vi "Init Tx - Data.vi"(7 "Data Access in":refnum<class "Data Access Engine.lvclass">, 8 "error in (no error)":errorcluster, 11 "Parameters":variant) -> (0 "error out":errorcluster, 3 "Tx Loop Data":T1, 5 "Data Access out":refnum<class "Data Access Engine.lvclass">)   [LabVIEW 2016, in "UDP-Custom-Device Engine.lvlib"]
uses:
  UDP-Custom-Device Engine.lvlib
  <vilib>/NI/NIVS Inline Async API/_Data Access Engine/Data Access Engine/Data Access Engine.lvclass
  Types/Engine - Tx Loop Data.ctl
  <vilib>/NI Veristand/VeriStand Data/Library/Byte Buffer/Byte Buffer.lvclass
  <vilib>/NI/NIVS Inline Async API/_Data Access Engine/Data Access Engine/Types/Read.DVR.ctl
  <vilib>/NI/NIVS Inline Async API/_Data Access Engine/Access Type Classes/Read/Read.lvclass
  <vilib>/NI Veristand/VeriStand Data/Library/Typedefs/Typedefs.Data Types.ctl
  Types/Engine - Data Conversion Config.ctl
  <vilib>/NI Veristand/VeriStand Data/Library/Byte Buffer/Byte Buffer.Mapping.ctl
  Shared/Types/Shared - Header Details.ctl
  Shared/Types/Shared - Tx.PacketInfo.ctl
  Shared/Types/Shared - Channel Data Type.ctl
  Shared/Types/Shared - Buffered.PacketInfo.ctl
  <vilib>/NI/NIVS Inline Async API/_Data Access Engine/Data Access Engine/Methods/Read.Lookup.vi
  Shared/UDP-Custom-Device Shared.lvlib
  <vilib>/NI Veristand/VeriStand Data/Library/VeriStand Data.lvlib
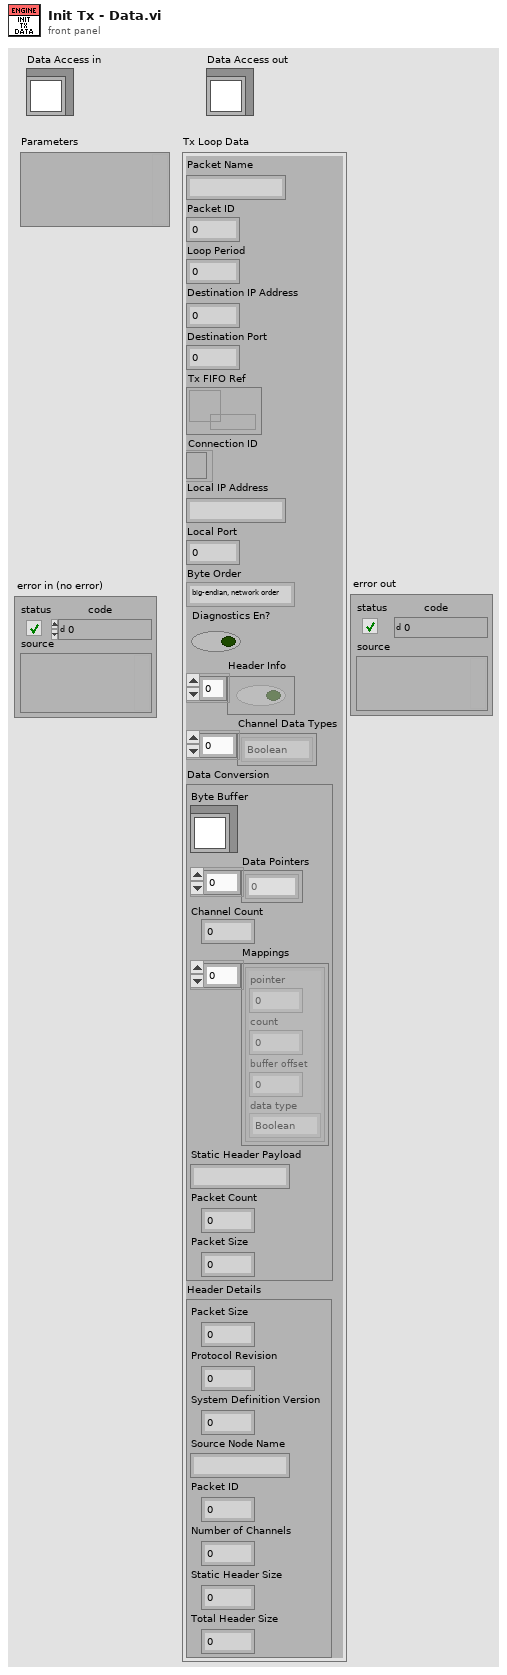
[diagram p1: front panel]
types:
  T1 = typedef "UDP-Custom-Device Engine.lvlib/Engine - Tx Loop Data.ctl" = cluster{"Packet Name":string, "Packet ID":i32, "Loop Period":u32, "Destination IP Address":u32, "Destination Port":u16, "Tx FIFO Ref":T2, "Connection ID":refnum<k16>, "Local IP Address":string, "Local Port":i32, "Byte Order":enum16{"big-endian, network order", "native, host order", "little-endian"}, "Diagnostics En?":bool, "Header Info":bool[], "Channel Data Types":T3[], "Data Conversion":T4, "Header Details":T6}
  T2 = typedef "Data Access Engine.lvlib/Data Access Engine.lvclass/Read.DVR.ctl" = refnum<data-value>
  T3 = typedef "VeriStand Data.lvlib/Typedefs.Data Types.ctl" = enum16{"Boolean", "Single", "Double", "I8", "I16", "I32", "I64", "U8", "U16", "U32", "U64"}
  T4 = typedef "UDP-Custom-Device Engine.lvlib/Engine - Data Conversion Config.ctl" = cluster{"Byte Buffer":refnum<class "Byte Buffer.lvclass">, "Data Pointers":u64[], "Channel Count":i32, "Mappings":T5[], "Static Header Payload":string, "Packet Count":dbl, "Packet Size":i32}
  T5 = typedef "VeriStand Data.lvlib/Byte Buffer.lvclass/Byte Buffer.Mapping.ctl" = cluster{"pointer":u64, "count":i32, "buffer offset":i32, "data type":T3}
  T6 = typedef "UDP-Custom-Device Shared.lvlib/Shared - Header Details.ctl" = cluster{"Packet Size":u16, "Protocol Revision":u8, "System Definition Version":u64, "Source Node Name":string, "Packet ID":u32, "Number of Channels":u32, "Static Header Size":u16, "Total Header Size":u16}
  T7 = typedef "UDP-Custom-Device Shared.lvlib/Shared - Tx.PacketInfo.ctl" = cluster{"Packet Name":string, "Packet ID":i32, "Decimation":u16, "Destination IP Address":string, "Destination Port":u16, "Local IP Address":string, "Local Port":u16, "Endianness":u16, "Diagnostics En?":bool, "Header Info":bool[], "PCL Period":u32, "Channel Data Types":T8[], "Header Details":T6, "Buffered Packet Info":T9}
  T8 = typedef "UDP-Custom-Device Shared.lvlib/Shared - Channel Data Type.ctl" = enum16{"Boolean", "Single", "Double", "I8", "I16", "I32", "I64", "U8", "U16", "U32", "U64"}
  T9 = typedef "UDP-Custom-Device Shared.lvlib/Shared - Buffered.PacketInfo.ctl" = cluster{"Buffer Size":u32, "External Buffer":bool, "Prepend Header":bool, "Is Buffered":bool}
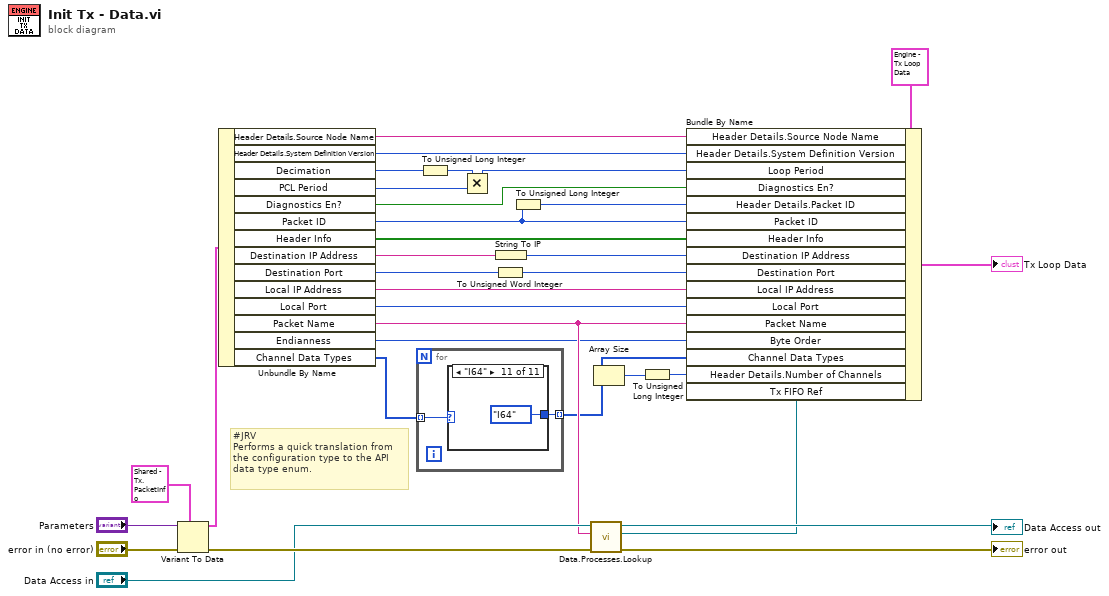
[diagram p0: block diagram]
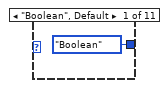
[diagram p2: hidden frame]
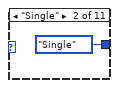
[diagram p3: hidden frame]
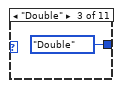
[diagram p4: hidden frame]
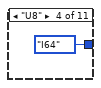
[diagram p5: hidden frame]
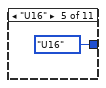
[diagram p6: hidden frame]
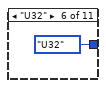
[diagram p7: hidden frame]
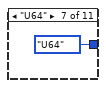
[diagram p8: hidden frame]
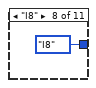
[diagram p9: hidden frame]
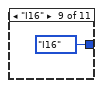
[diagram p10: hidden frame]
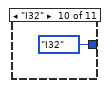
[diagram p11: hidden frame]
diagram:
  # "#JRV\nPerforms a quick translation from\nthe configuration type to the API\ndata type enum."
  n1 = Variant To Data(error in="error in (no error)", type=T7 {"Packet Name"="", "Packet ID"=0, "Decimation"=0, "Destination IP Address"="", "Destination Port"=0, "Local IP Address"="", "Local Port"=0, "Endianness"=0, "Diagnostics En?"=FALSE, "Header Info"=[], "PCL Period"=0, "Channel Data Types"=[], "Header Details"={"Packet Size"=0, "Protocol Revision"=0, "System Definition Version"=0, "Source Node Name"="", "Packet ID"=0, "Number of Channels"=0, "Static Header Size"=0, "Total Header Size"=0}, "Buffered Packet Info"={"Buffer Size"=0, "External Buffer"=FALSE, "Prepend Header"=FALSE, "Is Buffered"=FALSE}} ("Packet Info"), Variant="Parameters") -> (data=w31:T7, error out=w30:errorcluster)
  n2 = Unbundle By Name(w31) -> ("Header Details.Source Node Name"=w2:string, "Header Details.System Definition Version"=w1:u64, "Decimation"=w15:u16, "PCL Period"=w16:u32, "Diagnostics En?"=w18:bool, "Packet ID"=w8:i32, "Header Info"=w17:bool[], "Destination IP Address"=w10:string, "Destination Port"=w12:u16, "Local IP Address"=w22:string, "Local Port"=w21:u16, "Packet Name"=w23:string, "Endianness"=w19:u16, "Channel Data Types"=w13:T8[])
  n3 = for {
    tunnel: w13 -> [w35] mode=indexing
    tunnel: [w34] -> w6 mode=indexing
    n4 = case shown="\"I64\"" w35 {
      tunnel: [Typedefs.Data_Types."Boolean" ("data type") Typedefs.Data_Types."Single" ("data type") Typedefs.Data_Types."Double" ("data type") Typedefs.Data_Types."I64" ("data type") Typedefs.Data_Types."U16" ("data type") Typedefs.Data_Types."U32" ("data type") Typedefs.Data_Types."U64" ("data type") Typedefs.Data_Types."I8" ("data type") Typedefs.Data_Types."I16" ("data type") Typedefs.Data_Types."I32" ("data type") Typedefs.Data_Types."I64" ("data type")] -> w34
      frame "Boolean", Default {
      }
      frame "Single" {
      }
      frame "Double" {
      }
      frame "U8" {
      }
      frame "U16" {
      }
      frame "U32" {
      }
      frame "U64" {
      }
      frame "I8" {
      }
      frame "I16" {
      }
      frame "I32" {
      }
      frame "I64" {
      }
    }
  }
  n5 = To Unsigned Long Integer(number=w15) -> (unsigned 32bit integer=w3:u32)
  n6 = Multiply(x=w3, y=w16) -> (x*y=w14:u32)
  n7 = To Unsigned Word Integer(number=w12) -> (unsigned 16bit integer=w11:u16)
  n8 = String To IP(1:w10) -> (0:w9:u32)
  n9 = To Unsigned Long Integer(number=w8) -> (unsigned 32bit integer=w7:u32)
  n10 = call-poly <vilib>:"Data.Processes.Lookup.vi"("error in (no error)"=w30, "Name"=w23, "Data Access API in"="Data Access in") -> ("error out"=→"error out":errorcluster, "Ref"=w20:T2, "Data Access API out"=→"Data Access out":refnum<class "Data Access Engine.lvclass">)  [unwired: 5 in, 1 out]
  n11 = Array Size(array=w6) -> (size(s)=w5:i32)
  n12 = To Unsigned Long Integer(number=w5) -> (unsigned 32bit integer=w4:u32)
  n13 = Bundle By Name(cluster=T1 {"Packet Name"="", "Packet ID"=0, "Loop Period"=0, "Destination IP Address"=0, "Destination Port"=0, "Tx FIFO Ref"=refnum, "Connection ID"=refnum, "Local IP Address"="", "Local Port"=0, "Byte Order"=enum."big-endian, network order", "Diagnostics En?"=FALSE, "Header Info"=[], "Channel Data Types"=[], "Data Conversion"={"Byte Buffer"=refnum, "Data Pointers"=[], "Channel Count"=0, "Mappings"=[], "Static Header Payload"="", "Packet Count"=0.0, "Packet Size"=0}, "Header Details"={"Packet Size"=0, "Protocol Revision"=0, "System Definition Version"=0, "Source Node Name"="", "Packet ID"=0, "Number of Channels"=0, "Static Header Size"=0, "Total Header Size"=0}} ("Tx Loop Data"), "Header Details.Source Node Name"=w2, "Header Details.System Definition Version"=w1, "Loop Period"=w14, "Diagnostics En?"=w18, "Header Details.Packet ID"=w7, "Packet ID"=w8, "Header Info"=w17, "Destination IP Address"=w9, "Destination Port"=w11, "Local IP Address"=w22, "Local Port"=w21, "Packet Name"=w23, "Byte Order"=w19, "Channel Data Types"=w6, "Header Details.Number of Channels"=w4, "Tx FIFO Ref"=w20) -> (→"Tx Loop Data":T1)
